vi "Sequencer State Control.vi"(8 "error in (no error)":errorcluster, 10 "parameters in":T1, 11 "Sequencer Module runtime in":refnum<class "Sequencer Module runtime.lvclass">) -> (0 "error out":errorcluster, 2 "parameters out":T1, 3 "Sequencer Module runtime out":refnum<class "Sequencer Module runtime.lvclass">)   [LabVIEW 2015, in "Sequencer Module runtime.lvclass"]
uses:
  Sequencer Module runtime.lvclass
  <vilib>/NI/Tag Bus/table/data table.ctl
  Sequencer Module runtime.lvclass/Sequencer Module runtime.ctl
  Sequencer State Enum.ctl
  <vilib>/NI/Tag Bus/table/data table.lvlib
panel:
  # "Manual Input"
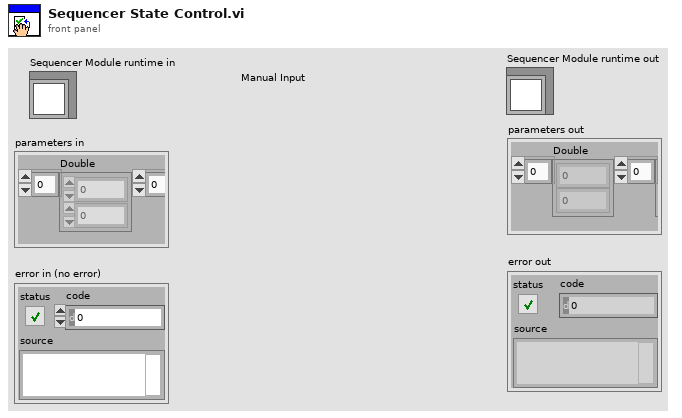
[diagram p1: front panel]
types:
  T1 = typedef "tag bus.lvlib/data table.lvlib/data table.ctl" = cluster{"Double":dbl[], "Single":sgl[], "I64":i64[], "I32":i32[], "I16":i16[], "I8":i8[], "U64":u64[], "U32":u32[], "U16":u16[], "U8":u8[], "Boolean":bool[], "String":string[], "Array of Double":cluster{"DBL Array":dbl[]}[], "Array of Single":cluster{"SGL Array":sgl[]}[], "Array of I64":cluster{"I64 Array":i64[]}[], "Array of I32":cluster{"I32 Array":i32[]}[], "Array of I16":cluster{"I16 Array":i16[]}[], "Array of I8":cluster{"I8 Array":i8[]}[], "Array of U64":cluster{"U64 Array":u64[]}[], "Array of U32":cluster{"U32 Array":u32[]}[], "Array of U16":cluster{"U16 Array":u16[]}[], "Array of U8":cluster{"U8 Array":u8[]}[], "Array of Boolean":cluster{"Boolean Array":bool[]}[], "Array of String":cluster{"String Array":string[]}[]}
  T2 = typedef "Sequencer Module runtime.lvclass/Sequencer Control.ctl" = cluster{"Start":bool, "Change Sequence":bool, "New Sequence":i32, "Pause":bool}
  T3 = typedef "Sequencer Module runtime.lvclass/Sequencer State Enum.ctl" = enum16{"Iddle", "Running", "Paused"}
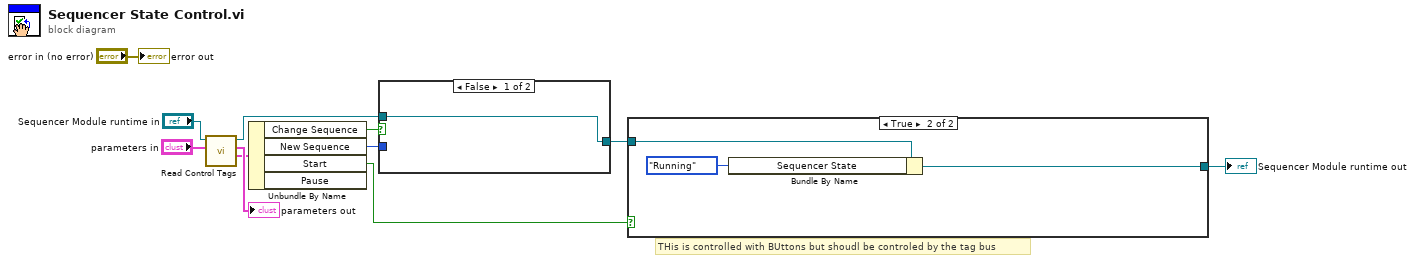
[diagram p0: block diagram]
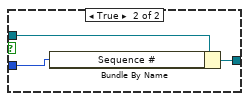
[diagram p3: hidden frame]
diagram:
  # "THis is controlled with BUttons but shoudl be controled by the tag bus"
  n1 = call "Read Control Tags.vi"("Paramaters  allocation in"="parameters in", "Sequencer Module runtime in"="Sequencer Module runtime in") -> ("Sequence Control"=w4:T2, "Parameters allocation out"=→"parameters out":T1, "Sequencer Module runtime out"=w7:refnum<class "Sequencer Module runtime.lvclass">)  [unwired: 7 in]
  n2 = Unbundle By Name(w4) -> ("Change Sequence"=w3:bool, "New Sequence"=w2:i32, "Start"=w1:bool)  [unwired: 1 out]
  n3 = case shown="False" w3 {
    tunnel: w7 -> [w12 w15]
    tunnel: w2 -> [_ w14]
    tunnel: [w12 w13] -> w10
    frame False {
    }
    frame True {
      n4 = Bundle By Name(cluster=w15, "Sequence #"=w14) -> (w13:refnum<class "Sequencer Module runtime.lvclass">)
    }
  }
  n5 = case shown="True" w1 {
    tunnel: w10 -> [w16 w19]
    tunnel: [w16 w18] -> w11
    frame False {
    }
    frame True {
      n6 = Bundle By Name(cluster=w19, "Sequencer State"=Sequencer_State_Enum."Running" ("Sequencer State.Sequencer State")) -> (w18:refnum<class "Sequencer Module runtime.lvclass">)
    }
  }
  "Sequencer Module runtime out" <- w11
  "error out" <- "error in (no error)"
